vi "Set Channel.vi"(8 "error in (no error)":errorcluster, 9 "Channel":refnum<class "CIFChannels.lvclass">, 10 "Channel Name":string, 11 "CIFChannelMng in":refnum<class "CIFChannelMng.lvclass">) -> (0 "error out":errorcluster, 3 "CIFChannelMng out":refnum<class "CIFChannelMng.lvclass">)   [LabVIEW 2021, in "CIFChannelMng.lvclass"]
uses:
  CIFChannelMng.lvclass
  CIFChannelMng.lvclass/CIFChannelMng.ctl
  CIFCore/Common/CIFCoreCommon.lvlib
  CIFClocks/Typedef/Errors.ctl
  <vilib>/Utility/miscctls.llb/LVMapReplaceAction.ctl
  CIFChannels/CIFChannels.lvclass
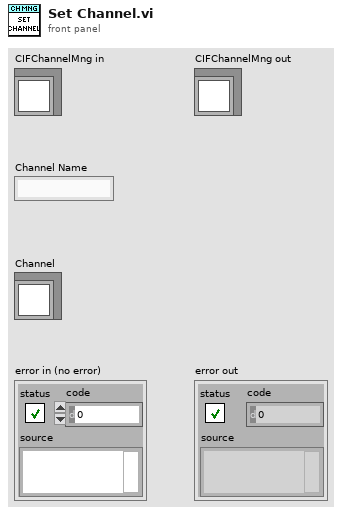
[diagram p1: front panel]
types:
  T1 = typedef "CIFCoreCommon.lvlib/Errors.ctl" = enum16{"Invalid Clock ID", "Long Sleep", "gRPC Server Not Found", "Config Parse", "Timestamp Wrap", "Delayed Execution", "Duplicate Channel", "Missing Channel", "Incorrect Type", "Unregistered Enum"}
  T2 = typedef "LVMapReplaceAction.ctl" = enum32{"Modify Entry only if found", "Add or Modify Entry", "Delete Entry"}
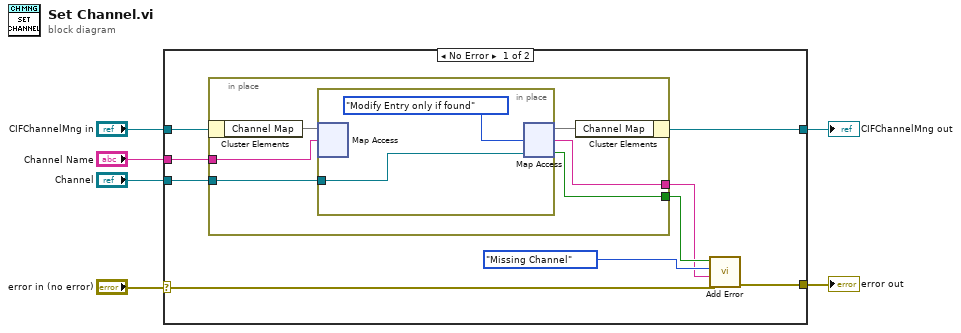
[diagram p0: block diagram]
diagram:
  n1 = case shown="No Error" "error in (no error)" {
    selector: "error in (no error)" -> [w8 w25]
    tunnel: [w13 w25] -> w6
    tunnel: [w15 w24] -> w5
    tunnel: "CIFChannelMng in" -> [w9 w24]
    tunnel: "Channel Name" -> [w7 _]
    tunnel: "Channel" -> [w12 _]
    frame No Error {
      n2 = in-place {
        in-place-border: w7 -> [w20]
        in-place-border: w12 -> [w18]
        in-place-border: [w17] -> w11
        in-place-border: [w16] -> w10
        n3 = in-place-cluster #1(w9) -> ("Channel Map"=w21:map{string, refnum<class "CIFChannels.lvclass">})
        n4 = in-place {
          in-place-border: w18 -> [w22]
          n5 = in-place-map #2(w21, w20) -> ()  [unwired: 1 in, 2 out]
          n6 = in-place-map #2(w22, LVMapReplaceAction."Modify Entry only if found" ("action")) -> (w19:map{string, refnum<class "CIFChannels.lvclass">}, w16:string, w17:bool)
        }
        n7 = in-place-cluster #1("Channel Map"=w19) -> (w15:refnum<class "CIFChannelMng.lvclass">)
      }
      n8 = call "Add Error.vi"("error in (no error)"=w8, "String to Append"=w10, "Error"=Errors."Missing Channel", "Insert Error"=w11) -> ("error out"=w13:errorcluster)  [unwired: 7 in]
    }
    frame Error {
    }
  }
  "error out" <- w6
  "CIFChannelMng out" <- w5
